vi "Launch Startup Clients.vi"(8 "error in":errorcluster, 11 "System in":refnum<class "System.lvclass">) -> (0 "error out":errorcluster, 3 "System out":refnum<class "System.lvclass">)   [LabVIEW 2014, in "System.lvclass"]
uses:
  System.lvclass
  Client_class/Client.lvclass
  Topic Child Classes/Launch Client/Launch Client.lvclass
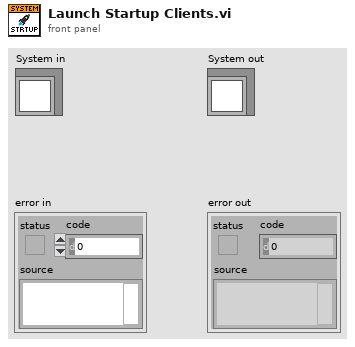
[diagram p1: front panel]
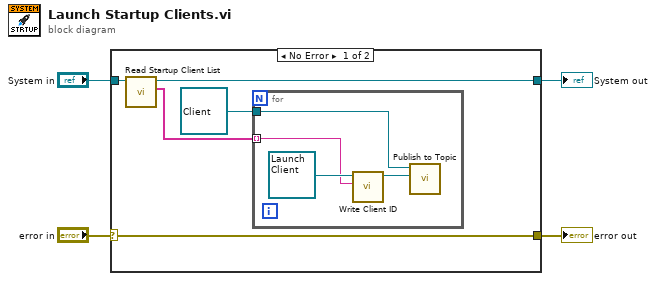
[diagram p0: block diagram]
diagram:
  n1 = case shown="No Error" "error in" {
    selector: "error in" -> [w8 w15]
    tunnel: [w8 w15] -> w3
    tunnel: [w7 w14] -> w1
    tunnel: "System in" -> [w9 w14]
    frame No Error {
      n2 = call-dynamic "Read Startup Client List.vi"("System in"=w9) -> ("Startup Client List"=w6:string[], "System out"=w7:refnum<class "System.lvclass">)  [unwired: 8 in, 1 out]
      n3 = for {
        tunnel: w6 -> [w11] mode=indexing
        tunnel: refnum<class "Client.lvclass"> refnum ("Client.lvclass") -> [w10]
        n4 = call-dynamic "Write Client ID.vi"("Client ID"=w11, "Launch Client in"=refnum<class "Launch Client.lvclass"> refnum ("Launch Client.lvclass")) -> ("Launch Client out"=w12:refnum<class "Launch Client.lvclass">)  [unwired: 8 in, 1 out]
        n5 = call-dynamic "Publish to Topic.vi"("Topic.lvclass"=w12, "Client in"=w10) -> ()  [unwired: 8 in, 2 out]
      }
    }
    frame Error {
    }
  }
  "error out" <- w3
  "System out" <- w1
